vi "leak_valve_analog.vi"(7 "read/write delay":dbl=0.5 caption="Delay Time (s)", 8 "desired_leak_rate (torr*l/s)":dbl, 9 "valve_pos_channel":tag="Dev3/ai4,Dev3/ai15", 10 "leak_control_channel":tag="Dev3/ao0") -> (1 "apparent_leak_rate":dbl=4.1159226100440096e-09, 2 "voltage_measured":dbl=0.0012441311525809389 format="%0.2f", 3 "voltage_applied":dbl)   [LabVIEW 2018]
uses:
  <vilib>/DAQmx/write.llb/DAQmx Write (Analog 1D DBL 1Chan NSamp).vi
  <vilib>/DAQmx/read.llb/DAQmx Read (Analog 2D DBL NChan NSamp).vi
  <vilib>/Analysis/baseanly.llb/Mean (DBL).vi
  <vilib>/Utility/file.llb/Read Delimited Spreadsheet (DBL).vi
  <vilib>/DAQmx/create/channels.llb/DAQmx Create Channel (AO-Voltage-Basic).vi
  <vilib>/DAQmx/miscellaneous.llb/DAQmx Fill In Error Info.vi
  <vilib>/DAQmx/create/channels.llb/DAQmx Create Channel (AI-Voltage-Basic).vi
  <vilib>/Analysis/NI_AALBase.lvlib
  <vilib>/gmath/NI_Gmath.lvlib
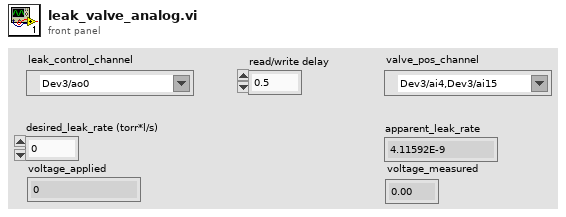
[diagram p1: front panel]
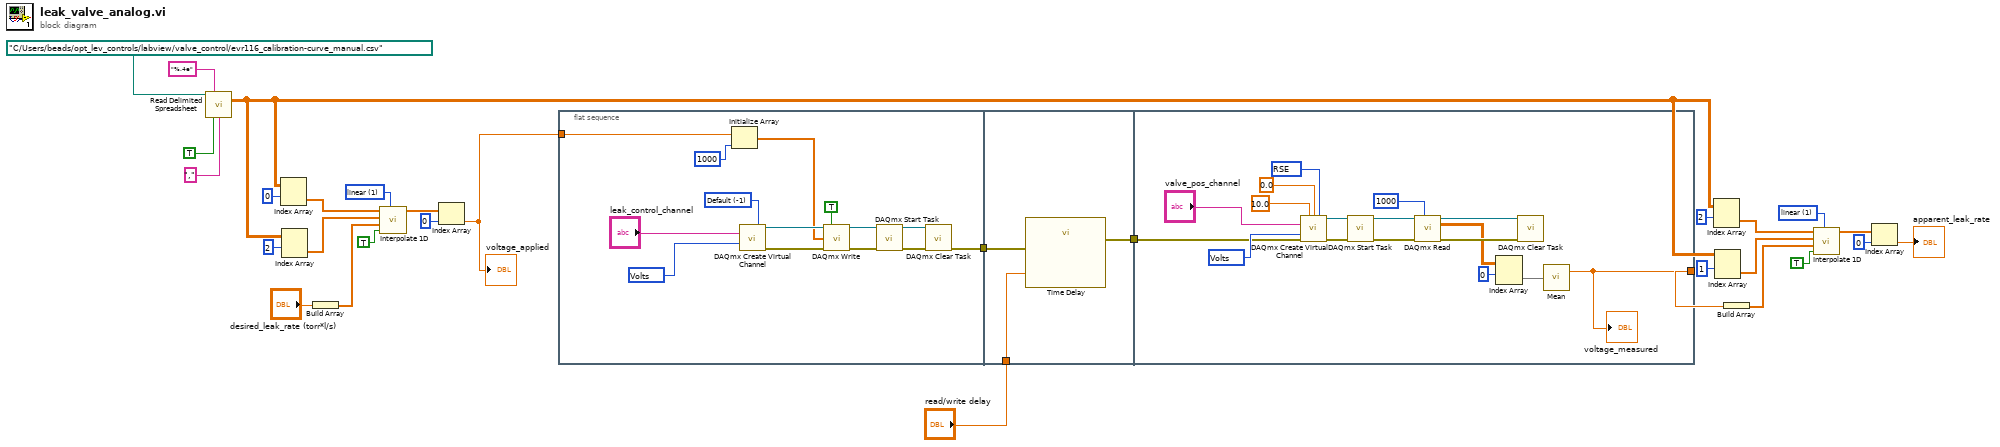
[diagram p0: block diagram]
diagram:
  w5 = 1 items=["nearest", "linear", "spline", "cubic Hermite", "Lagrange"] ("method")
  w20 = 1 items=["nearest", "linear", "spline", "cubic Hermite", "Lagrange"] ("method")
  n1 = call-poly <vilib>:"Read Delimited Spreadsheet.vi"("file path (dialog if empty)"=path "C:/Users/beads/opt_lev_controls/labview/valve_control/evr116_calibration-curve_manual.csv", "format (%.3f)"="%.4e", "transpose? (F)"=TRUE, "delimiter (\\t)"="," ("delimiter (\\t)")) -> ("all rows"=w24:dbl[][])  [unwired: 6 in, 5 out]
  n2 = Index Array(array=w24, index (row)=0) -> (element=w19:dbl[])  [unwired: 1 in]
  n3 = Index Array(array=w24, index (row)=2) -> (element=w18:dbl[])  [unwired: 1 in]
  n4 = Build Array("desired_leak_rate (torr*l/s)") -> (w16:dbl[])
  n5 = call <vilib>:"Interpolate 1D.vi"("method"=w20, "X is monotonic"=TRUE, "xi"=w16, "X"=w18, "Y"=w19) -> ("yi"=w14:dbl[])  [unwired: 4 in, 2 out]
  n6 = Index Array(array=w14, index=0) -> (element=w23:dbl)
  "voltage_applied" <- w23
  n7 = flat-sequence {
    tunnel: [w32] -> w30
    tunnel: w23 -> [w31]
    tunnel: w30 -> [w47]
    tunnel: [w46] -> w29
    tunnel: "read/write delay" -> [w45]
    tunnel: w29 -> [w49]
    tunnel: [w48] -> w6
    frame #0 {
      w42 = -1 items=["Default"=-1, "RSE"=10083, "Differential"=10106, "Pseudodifferential"=12529] ("output terminal configuration")
      w43 = 10348 items=["Volts"=10348, "From Custom Scale"=10065] ("units")
      n8 = Initialize Array(w31, 1000 ("dimension size")) -> (w38:dbl[])
      n9 = call-poly <vilib>:"DAQmx Create Virtual Channel.vi"("output terminal configuration"=w42, "physical channels"="leak_control_channel", "units"=w43) -> ("task out"=w41:refnum<k21>, "error out"=w40:errorcluster)  [unwired: 11 in]
      n10 = call-poly <vilib>:"DAQmx Write.vi"("task/channels in"=w41, "auto start"=TRUE, "data"=w38, "error in"=w40) -> ("task out"=w37:refnum<k21>, "error out"=w36:errorcluster)  [unwired: 9 in, 1 out]
      n11 = call <vilib>:"DAQmx Start Task.vi"("task/channels in"=w37, "error in"=w36) -> ("task out"=w35:refnum<k21>, "error out"=w34:errorcluster)  [unwired: 12 in]
      n12 = call <vilib>:"DAQmx Clear Task.vi"("task in"=w35, "error in"=w34) -> ("error out"=w32:errorcluster)  [unwired: 13 in]
    }
    frame #1 {
      n13 = call "Time Delay"("error in (no error)"=w47, "Delay Time (s)"=w45) -> ("error out"=w46:errorcluster)  [unwired: 9 in]
    }
    frame #2 {
      w51 = 10083 items=["default"=-1, "RSE"=10083, "NRSE"=10078, "Differential"=10106, "Pseudodifferential"=12529] ("input terminal configuration")
      w50 = 10348 items=["Volts"=10348, "From Custom Scale"=10065] ("units")
      n14 = call-poly <vilib>:"DAQmx Create Virtual Channel.vi"("maximum value"=10.0, "minimum value"=0.0, "input terminal configuration"=w51, "physical channels"="valve_pos_channel", "units"=w50, "error in"=w49) -> ("task out"=w58:refnum<k21>, "error out"=w62:errorcluster)  [unwired: 8 in]
      n15 = call <vilib>:"DAQmx Start Task.vi"("task/channels in"=w58, "error in"=w62) -> ("task out"=w59:refnum<k21>, "error out"=w63:errorcluster)  [unwired: 12 in]
      n16 = call-poly <vilib>:"DAQmx Read.vi"("task/channels in"=w59, "number of samples per channel"=1000, "error in"=w63) -> ("task out"=w57:refnum<k21>, "data"=w60:dbl[][], "error out"=w64:errorcluster)  [unwired: 10 in]
      n17 = Index Array(array=w60, index (row)=0) -> (element=w61:dbl[])  [unwired: 1 in]
      n18 = call <vilib>:"DAQmx Clear Task.vi"("task in"=w57, "error in"=w64) -> ()  [unwired: 13 in, 1 out]
      n19 = call-poly <vilib>:"Mean.vi"("X"=w61) -> ("mean"=w48:dbl)  [unwired: 1 out]
      "voltage_measured" <- w48
    }
  }
  n20 = Index Array(array=w24, index (row)=2) -> (element=w8:dbl[])  [unwired: 1 in]
  n21 = Index Array(array=w24, index (row)=1) -> (element=w9:dbl[])  [unwired: 1 in]
  n22 = Build Array(w6) -> (w10:dbl[])
  n23 = call <vilib>:"Interpolate 1D.vi"("method"=w5, "X is monotonic"=TRUE, "xi"=w10, "X"=w9, "Y"=w8) -> ("yi"=w11:dbl[])  [unwired: 4 in, 2 out]
  n24 = Index Array(array=w11, index=0) -> (element=→"apparent_leak_rate":dbl)
